vi "Measure Jitter.vi"(6 "Target Data":T1, 8 "error in (no error)":errorcluster, 9 "No. Periods":u32, 10 "Channel":T2, 11 "MSOX6004 in":refnum<class "MSOX6004.lvclass">) -> (0 "error out":errorcluster, 2 "Jitter":dbl, 3 "MSOX6004 out":refnum<class "MSOX6004.lvclass">)   [LabVIEW 2018, in "MSOX6004.lvlib" / "MSOX6004.lvclass"]
uses:
  MSOX6004.lvclass
  PPLs/Oscilloscope/Parent/Oscilloscope.lvlibp/Custom Controls/Analog Channels.ctl
  PPLs/Oscilloscope/Parent/Oscilloscope.lvlibp/Custom Controls/Target Data.ctl
  MSOX6004.lvclass/MSOX6004.ctl
  <instrlib>/Keysight InfiniiVision/Keysight InfiniiVision.lvlib
  PPLs/Oscilloscope/Parent/Oscilloscope.lvlibp
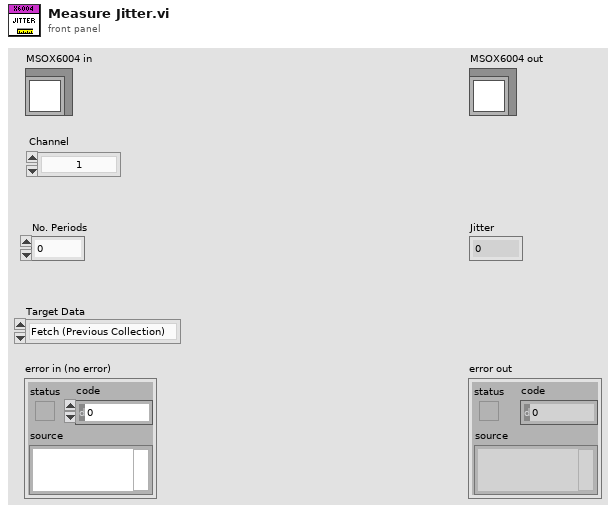
[diagram p1: front panel]
types:
  T1 = typedef "Oscilloscope.lvlibp/Target Data.ctl" = enum16{"Fetch (Previous Collection)", "Measure (New Collection)"}
  T2 = typedef "Oscilloscope.lvlibp/Analog Channels.ctl" = enum16{"1", "2", "3", "4", "5", "6", "7", "8", "9", "10", "11", "12", "13", "14", "15", "16"}
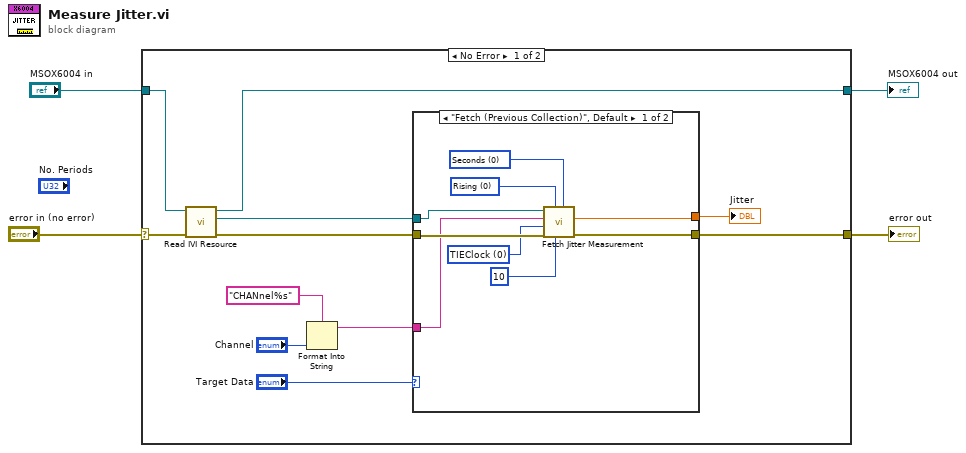
[diagram p0: block diagram]
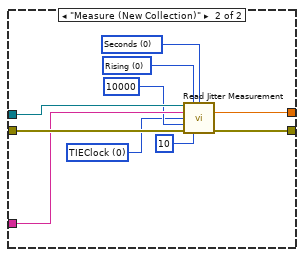
[diagram p2: hidden frame]
diagram:
  n1 = case shown="No Error" "error in (no error)" {
    selector: "error in (no error)" -> [w15 w36]
    tunnel: [w8 w36] -> w3
    tunnel: [w13 w35] -> w2
    tunnel: "MSOX6004 in" -> [w14 w35]
    frame No Error {
      n2 = call "Read IVI Resource.vi"("error in (no error)"=w15, "MSOX6004 in"=w14) -> ("error out"=w9:errorcluster, "IVI Resource"=w6:refnum<k15>, "MSOX6004 out"=w13:refnum<class "MSOX6004.lvclass">)  [unwired: 7 in]
      n3 = Format Into String(format string="CHANnel%s", "Channel") -> (resulting string=w7:string)  [unwired: 2 in, 1 out]
      n4 = case shown="\"Fetch (Previous Collection)\", Default" "Target Data" {
        tunnel: w9 -> [w24 w34]
        tunnel: [w23 w33] -> w8
        tunnel: w7 -> [w20 w32]
        tunnel: w6 -> [w21 w31]
        tunnel: [w22 w27] -> w5
        frame "Fetch (Previous Collection)", Default {
          w16 = 0 items=["Seconds", "Interval"] ("Unit (Seconds)")
          w17 = 0 items=["Rising", "Falling", "Both"] ("Slope (Rising)")
          w19 = 0 items=["TIEClock", "TIEData", "NCJitter", "NPeriod", "CTCNWidth", "CTCPWidth"] ("MeasFunction (TIEClock)")
          n5 = call <instrlib>:"Fetch Jitter Measurement.vi"("Unit (Seconds)"=w16, "NumberOfPeriods (1)"=10, "Slope (Rising)"=w17, "error in (no error)"=w24, "MeasFunction (TIEClock)"=w19, "Measurement"=w20, "instrument handle"=w21) -> ("error out"=w23:errorcluster, "Result"=w22:dbl)  [unwired: 2 in, 1 out]
        }
        frame "Measure (New Collection)" {
          w25 = 0 items=["Seconds", "Interval"] ("Unit (Seconds)")
          w26 = 0 items=["Rising", "Falling", "Both"] ("Slope (Rising)")
          w28 = 0 items=["TIEClock", "TIEData", "NCJitter", "NPeriod", "CTCNWidth", "CTCPWidth"] ("MeasFunction (TIEClock)")
          n6 = call <instrlib>:"Read Jitter Measurement.vi"("instrument handle"=w31, "Slope (Rising)"=w26, "Unit (Seconds)"=w25, "Measurement"=w32, "MeasFunction (TIEClock)"=w28, "MaxTimeMilliseconds"=10000, "error in (no error)"=w34, "NumberOfPeriods"=10) -> ("Result"=w27:dbl, "error out"=w33:errorcluster)  [unwired: 5 in, 1 out]
        }
      }
      "Jitter" <- w5
    }
    frame Error {
    }
  }
  "error out" <- w3
  "MSOX6004 out" <- w2
